vi "Obtain UIM.vi"(8 "Error In":errorcluster) -> (0 "Error Out":errorcluster, 3 "UIM Handle":refnum<data-value>)   [LabVIEW 2015, in "UIM.lvclass"]
doc: "Obtain the session of the UIM. The path to UIP folder defines the location of the plugin UIPs to be loaded when the UIM is initialized. Only the <b>loaded UIPs and the default UIPs</b> will be used in the current session of UIM. This means only the handled properties of controls and indicators will be saved and restored in states.\n\nIf this method is called on a system that does not have any plugins installed in the default folder, it will return without any UIPs loaded. In this case you need to specify your own UIPs before working with states.\n\nIf you would like to work with more or less UIPs, you should use the UIP methods to load or remove them."
uses:
  UIM.lvclass
  UIM.lvclass/UIM.ctl
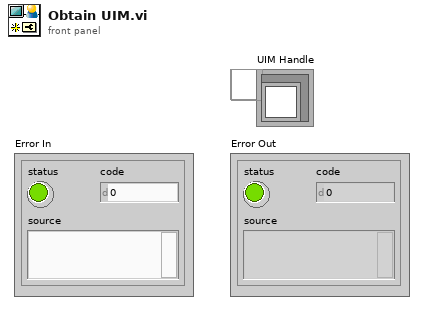
[diagram p1: front panel]
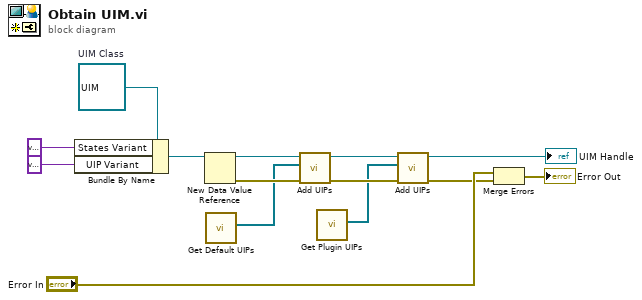
[diagram p0: block diagram]
diagram:
  w12 = refnum<class "UIM.lvclass"> refnum  # UIM Class
  n1 = Bundle By Name(cluster=w12, "States Variant"=variant, "UIP Variant"=variant) -> (w11:refnum<class "UIM.lvclass">)
  n2 = New Data Value Reference(data value=w11) -> (data value reference=w9:refnum<data-value>, error out=w10:errorcluster)  [unwired: 1 in]
  n3 = call "Get Default UIPs.vi"() -> ("UIPs"=w6:refnum<class "UIP.lvclass">[])  [unwired: 11 in]
  n4 = call "Add UIPs.vi"("Error In"=w10, "UIPs"=w6, "UIM In"=w9) -> ("Error Out"=w4:errorcluster, "UIM Out"=w5:refnum<data-value>)  [unwired: 7 in]
  n5 = call "Get Plugin UIPs.vi"() -> ("UIPs"=w3:refnum<class "UIP.lvclass">[])  [unwired: 11 in]
  n6 = call "Add UIPs.vi"("Error In"=w4, "UIPs"=w3, "UIM In"=w5) -> ("Error Out"=w1:errorcluster, "UIM Out"=→"UIM Handle":refnum<data-value>)  [unwired: 7 in]
  n7 = Merge Errors("Error In", w1) -> (→"Error Out":errorcluster)
